vi "PPFS_SIM_SIM_MODULE_INIT.vi"(3 "Module Index":i32, 4 "SwerveRadiansPerCount":dbl=1.0, 5 "Drive PWM Channel":T2, 6 "DriveDistPerCount":dbl=1.0, 7 "Swerve PWM Channel":T2, 8 "Swerve B Channel":T1, 9 "Swerver A Channel":T1, 10 "Drive B Channel":T1, 11 "Drive A channel":T1) -> ()   [LabVIEW 2023]
uses:
  <vilib>/Rock Robotics/SystemInterfaces/DIO/FPGA_DIOChannel.ctl
  <vilib>/Rock Robotics/SystemInterfaces/DIO/FPGA_DIOPWMChannel.ctl
  PPFS_SIM_SIM_Globals.vi
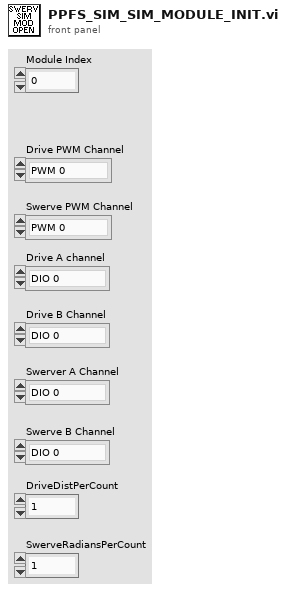
[diagram p1: front panel]
types:
  T1 = typedef "FPGA_DIOChannel.ctl" = enum8{"DIO 0", "DIO 1", "DIO 2", "DIO 3", "DIO 4", "DIO 5", "DIO 6", "DIO 7", "DIO 8", "DIO 9", "DIO MXP 0", "DIO MXP 1", "DIO MXP 2", "DIO MXP 3", "DIO MXP 4", "DIO MXP 5", "DIO MXP 6", "DIO MXP 7", "DIO MXP 8", "DIO MXP 9", "DIO MXP 10", "DIO MXP 11", "DIO MXP 12", "DIO MXP 13", "DIO MXP 14", "DIO MXP 15", "SPI Port CS1", "SPI Port CS2", "SPI Port CS3", "SPI Port MISO", "SPI Port MOSI", "Invalid"}
  T2 = typedef "FPGA_DIOPWMChannel.ctl" = enum8{"PWM 0", "PWM 1", "PWM 2", "PWM 3", "PWM 4", "PWM 5", "PWM 6", "PWM 7", "PWM 8", "PWM 9", "PWM MXP 0", "PWM MXP 1", "PWM MXP 2", "PWM MXP 3", "PWM MXP 4", "PWM MXP 5", "PWM MXP 6", "PWM MXP 7", "PWM MXP 8", "PWM MXP 9", "Invalid"}
  T3 = cluster{"Swerve Device Index":i32, "Drive Device Index":i32, "Drive DistPerzcount":dbl, "SwerveRadPerCount":dbl}[]
  T4 = typedef "PPFS_DRIVE_MODULE_TYPDEF.ctl" = cluster{"SwervDrive":T5, "SwerveSwerve":T5}
  T5 = typedef "WPI_MotorControlDeviceRef.ctl" = cluster{"DeviceStatus":errorcluster, "Type":T6, "PWM":cluster{"PWM Channel":T2, "DeadBand":T7}, "CAN":cluster{"Device Number":u8, "SetOutput VI Ref":variant, "GetOutput VI Ref":variant, "Enable VI Ref":variant, "Disable VI Ref":variant, "Data":variant}, "Invert":bool, "DIO PWM":cluster{"PWM \"Enable\" Channel":T2, "DIOChannel":T1, "PWM Rate":dbl}}
  T6 = typedef "WPI_MotorControlType.ctl" = enum16{"PWM", "CAN", "DIO PWM"}
  T7 = typedef "WPI_PWMDeadband.ctl" = cluster{"Name":string, "maxPositivePwm":i32, "minPositivePwm":i32, "centerPwm":i32, "maxNegativePwm":i32, "minNegativePwm":i32, "angularRange":u16}
  T8 = cluster{"Swerve Device Index":i32, "Drive Device Index":i32, "Drive DistPerzcount":dbl, "SwerveRadPerCount":dbl}
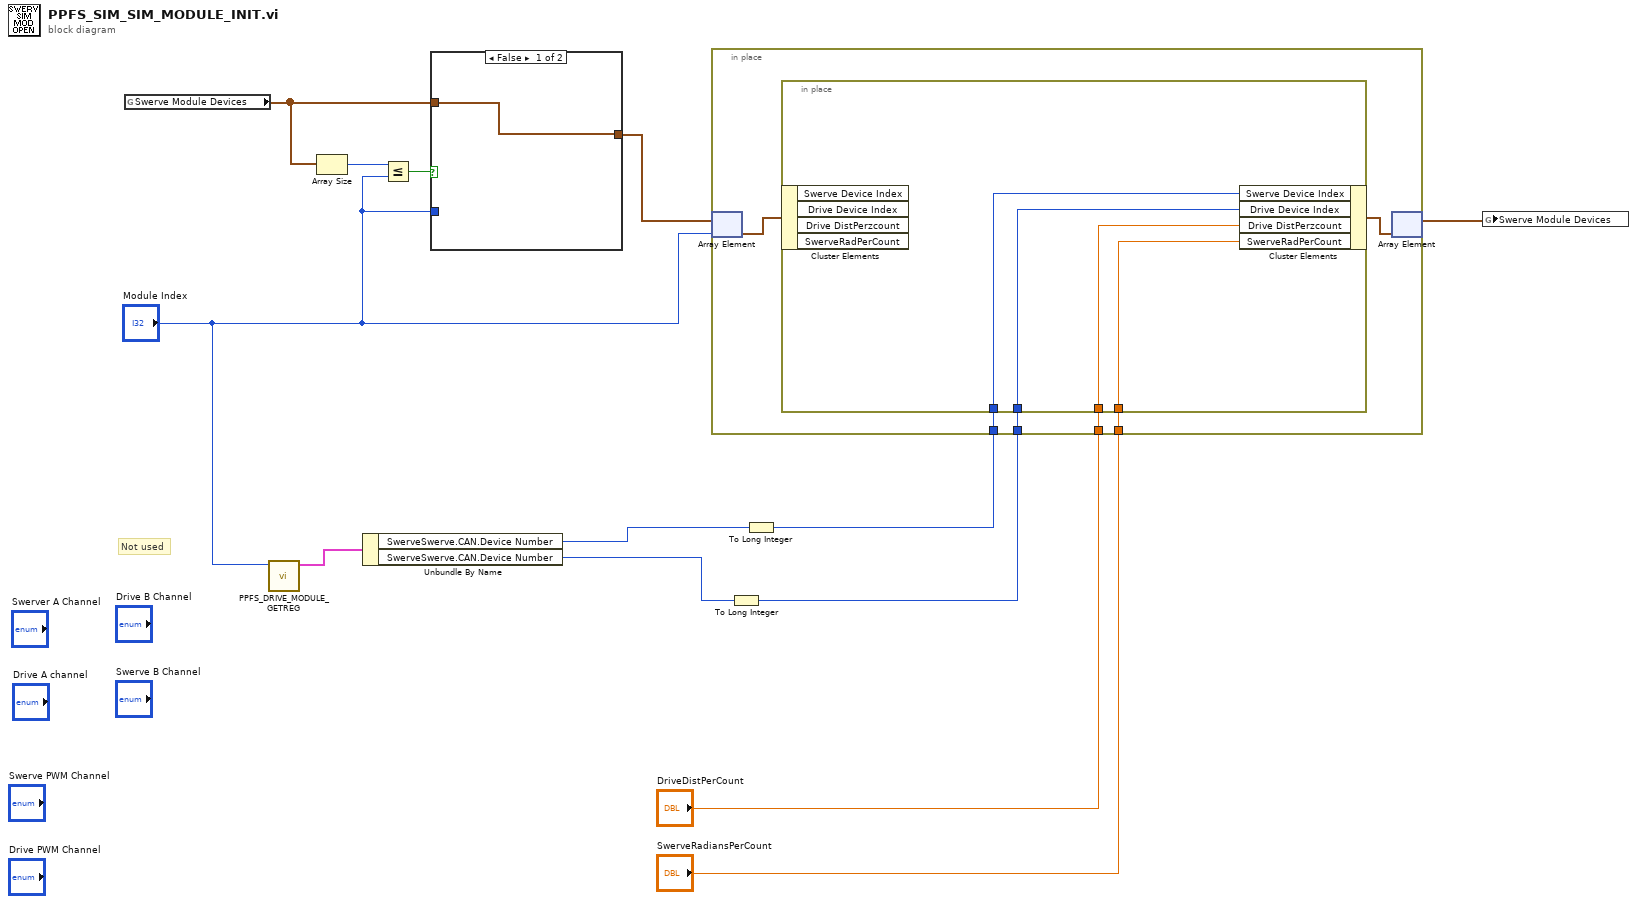
[diagram p0: block diagram]
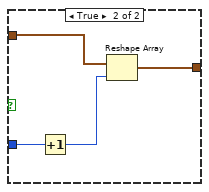
[diagram p2: hidden frame]
diagram:
  # "Not used"
  n1 = global read "PPFS_SIM_SIM_Globals.vi" "Swerve Module Devices"() -> (w8:T3)
  n2 = call "PPFS_DRIVE_MODULE_GETREG.vi"("Suffix"="Module Index") -> ("Swerve Module TypDef"=w6:T4)  [unwired: 10 in]
  n3 = Array Size(array=w8) -> (size(s)=w10:i32)
  n4 = Unbundle By Name(w6) -> ("SwerveSwerve.CAN.Device Number"=w4:u8, "SwerveSwerve.CAN.Device Number"=w3:u8)
  n5 = Less Or Equal?(x=w10, y="Module Index") -> (x <= y?=w9:bool)
  n6 = case shown="False" w9 {
    tunnel: w8 -> [w14 w16]
    tunnel: "Module Index" -> [_ w18]
    tunnel: [w14 w15] -> w7
    frame False {
    }
    frame True {
      n7 = Increment(x=w18) -> (x+1=w17:i32)
      n8 = Reshape Array(w16, w17) -> (w15:T3)
    }
  }
  n9 = To Long Integer(number=w3) -> (32bit integer=w1:i32)
  n10 = To Long Integer(number=w4) -> (32bit integer=w2:i32)
  n11 = in-place {
    in-place-border: w2 -> [w23]
    in-place-border: w1 -> [w22]
    in-place-border: "DriveDistPerCount" -> [w20]
    in-place-border: "SwerveRadiansPerCount" -> [w19]
    n12 = in-place-array #1(w7, "Module Index") -> (w24:T8)
    n13 = in-place {
      in-place-border: w23 -> [w28]
      in-place-border: w22 -> [w27]
      in-place-border: w20 -> [w26]
      in-place-border: w19 -> [w25]
      n14 = in-place-cluster #2(w24) -> ()  [unwired: 4 out]
      n15 = in-place-cluster #2("Swerve Device Index"=w28, "Drive Device Index"=w27, "Drive DistPerzcount"=w26, "SwerveRadPerCount"=w25) -> (w21:T8)
    }
    n16 = in-place-array #1(w21) -> (w13:T3)  [unwired: 1 out]
  }
  n17 = global write "PPFS_SIM_SIM_Globals.vi" "Swerve Module Devices"(w13) -> ()
